vi "Helium Fridge Cool-Down.vi"() -> ()   [LabVIEW 2014]
uses:
  <vilib>/Analysis/8numeric.llb/1D Numeric Integration.vi
  <vilib>/express/express shared/transition.llb/Dynamic To Waveform Array.vi
  <vilib>/express/express signal manip/GetorSetDDTAttributes/Set DDT Attributes/SetT0.vi
  <vilib>/express/express shared/transition.llb/Waveform Array To Dynamic.vi
  <vilib>/express/express signal manip/GetorSetDDTAttributes/Set DDT Attributes/Set DDT Properties.xnode
  <vilib>/Analysis/NI_AALPro.lvlib
panel:
  in  "Submit":bool
  out "Is Flashing":bool
  in  "Error Beat":bool
  in  "Clear":bool
  in  "Comment":string
  out "Heartbeat":bool
  out "Most Recent Error":string
  out "Baseline Subtracted Integral vs. Time":dbl(graph)
  out "Time of Last Baseline":string
  out "Baseline":dbl[](array[numeric])
  in  "Baseline Subtract":bool
  in  "Get Baseline":bool
  out "Recording":bool
  out "Time of Last Recording":string
  in  "Record \nNMR Sweeps":bool
  in  "Depth/Div\n(kHz)":dbl=10.0
  in  "Central Freq. \n(MHz)":dbl=13.0
  in  "stop (F)":bool caption="Triangle Wave"
  in  "Triangle Wave\nRate (Hz)":dbl=0.3
  out "Time Elapsed \nDuring Sweeps (s)":dbl
  out "Lab Time":string
  out "Most Recent Error (NMR)":string
  out "Last Sweep Start Time":string
  out "Most Recent Error (Temp)":string
  out "Last Measurement Taken":string
  out "VI Start Time":string
  in  "Time Between\nTemp Ponts (s)":dbl=30.0
  out "Temp":bool
  out "NMR":bool
  in  "stop":bool
  out "Input Triangle Wave":dynamicdata(graph)
  out "Modulator":dynamicdata(graph)
  out "NMR":cluster{"Y":dbl[], "Y":dbl[]}[](graph)
  in  "# of Sweeps":dbl=1.0
  out "Resistance Strip Chart":dynamicdata(graph)
  out "Temperature Strip Chart":dynamicdata(graph)
  in  "Heartbeat":bool
  in  "Temp Strip Chart":bool
  out "Errors":bool
  in  "Silence Flashing":bool
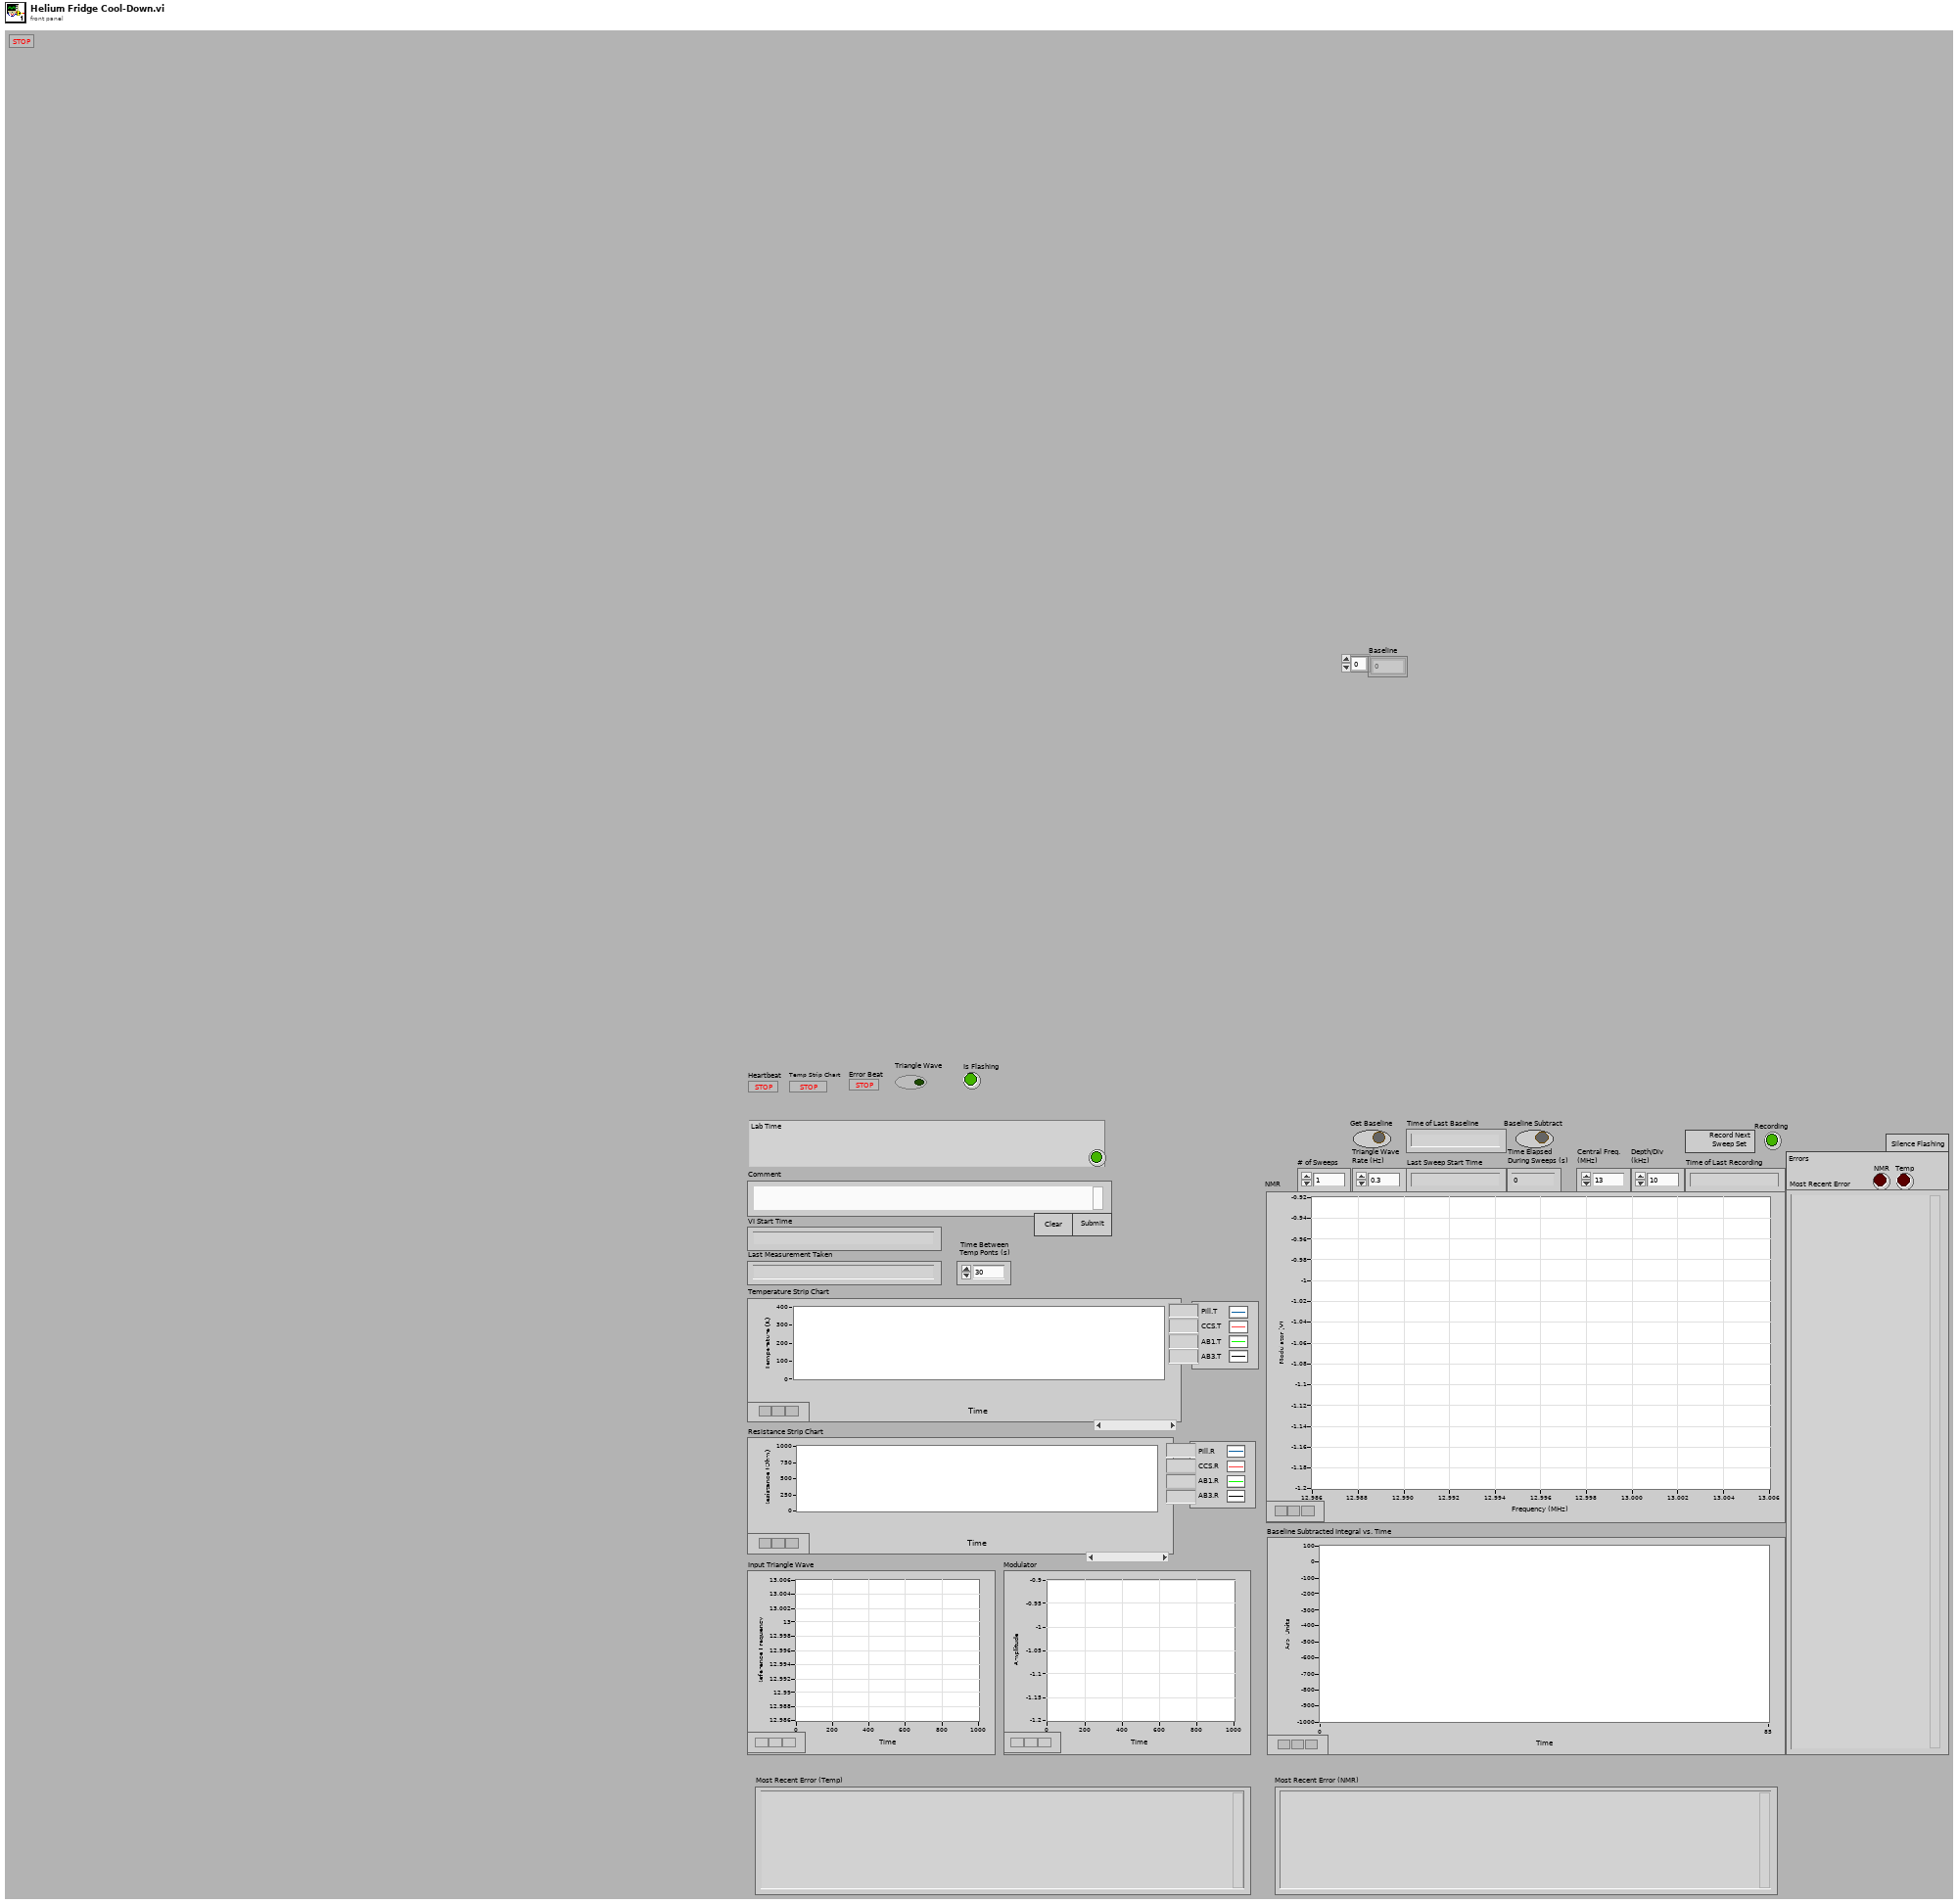
[diagram p1: front panel]
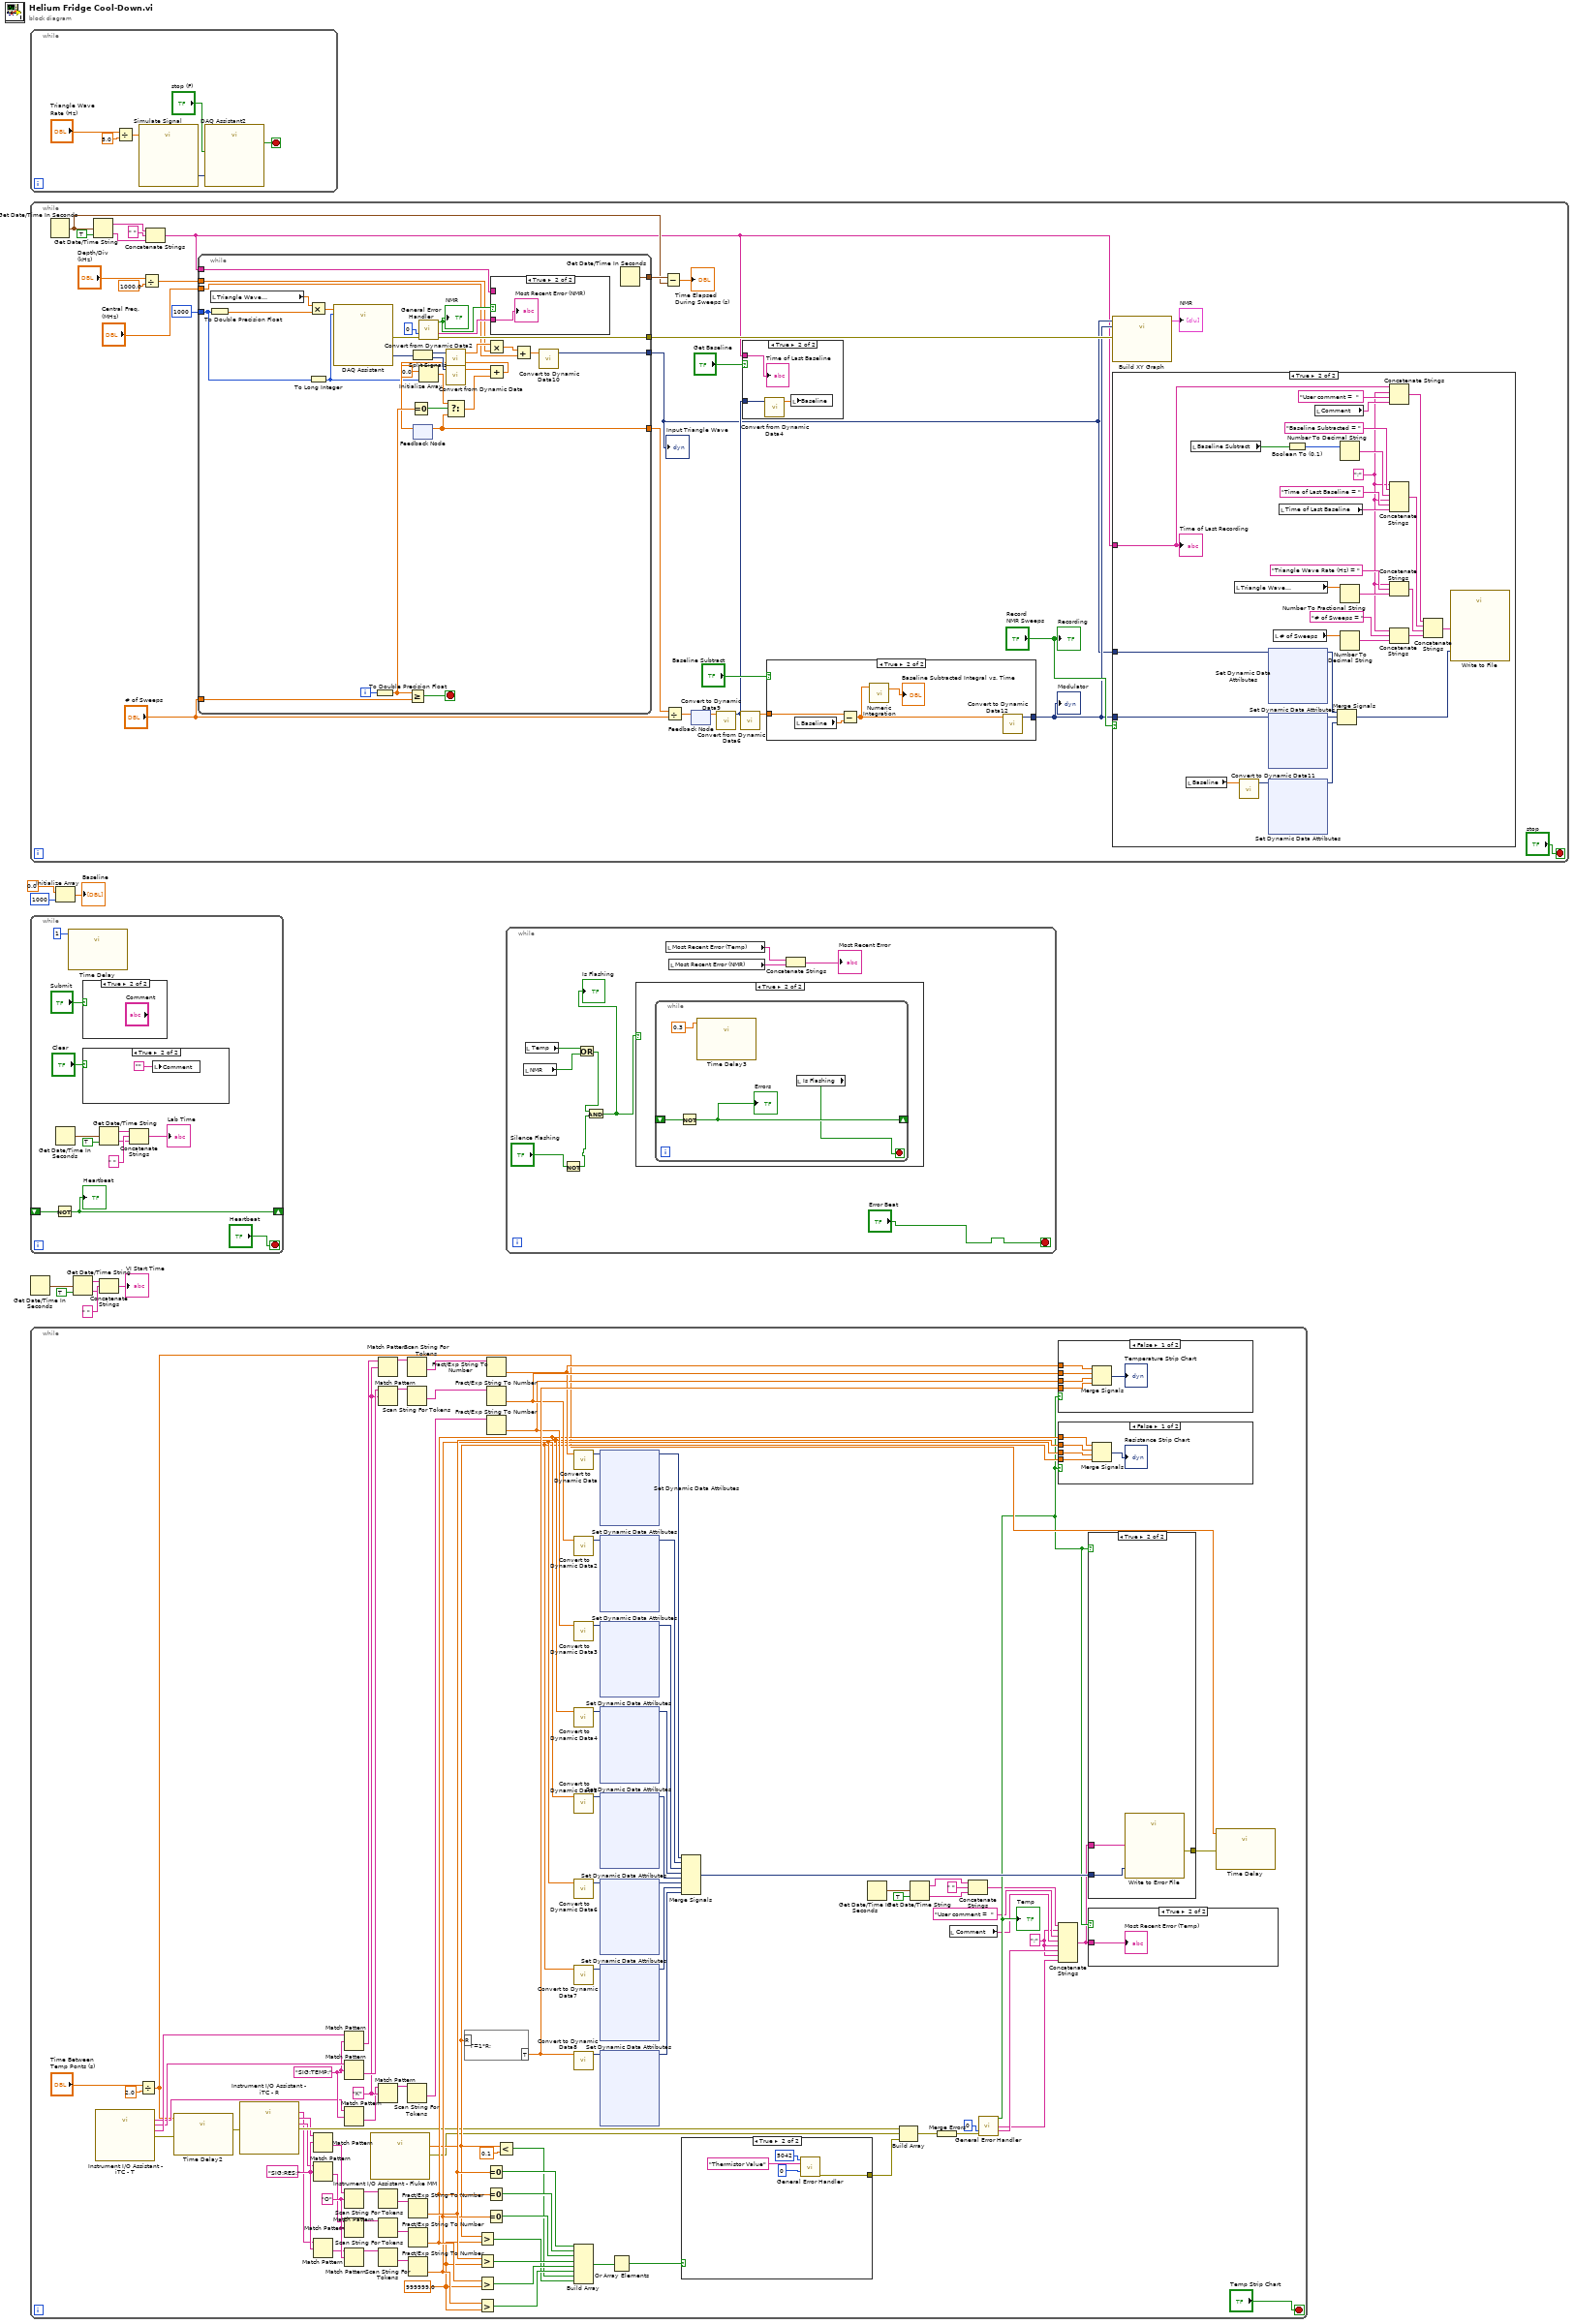
[diagram p0: block diagram]
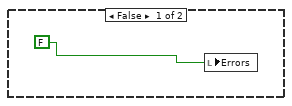
[diagram p2: hidden frame]
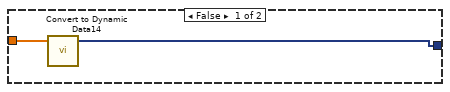
[diagram p3: hidden frame]
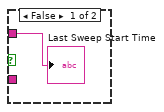
[diagram p6: hidden frame]
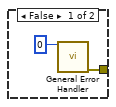
[diagram p9: hidden frame]
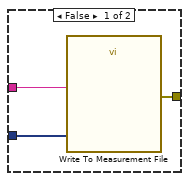
[diagram p12: hidden frame]
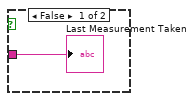
[diagram p13: hidden frame]
diagram:
  n1 = while {
    stop <- w14 stop-if-true
    n2 = Divide(x="Triangle Wave\nRate (Hz)", y=5.0) -> (x/y=w10:dbl)
    n3 = call "Simulate Signal"("Frequency"=w10) -> ("Triangle"=w13:dynamicdata)  [unwired: 13 in, 1 out]
    n4 = call "DAQ Assistant2"("data"=w13, "stop (F)"="stop (F)") -> ("stopped"=w14:bool)  [unwired: 15 in, 2 out]
  }
  n5 = while {
    stop <- "stop" stop-if-true
    n6 = Get Date/Time In Seconds() -> (seconds since 1Jan1904=w30:timestamp)
    n7 = Get Date/Time String(seconds (now)=w30, want seconds? (F)=TRUE) -> (date string=w33:string, time string=w35:string)  [unwired: 1 in]
    n8 = Divide(x="Depth/Div\n(kHz)", y=1000.0) -> (x/y=w24:dbl)
    n9 = Concatenate Strings(w33, " ", w35) -> (w16:string)
    n10 = while {
      tunnel: "# of Sweeps" -> [w163]
      tunnel: 1000 -> [w143]
      tunnel: [w156] -> w39
      tunnel: w16 -> [w150]
      tunnel: [w149] -> w31
      tunnel: [w147] -> w28
      tunnel: w24 -> [w140]
      tunnel: "Central Freq. \n(MHz)" -> [w138]
      tunnel: [w136] -> w17
      i -> [w164]
      stop <- w155 stop-if-true
      n11 = To Double Precision Float(number=w143) -> (double precision float=w144:dbl)
      n12 = local read "Triangle Wave\nRate (Hz)"() -> (w146:dbl)
      n13 = Multiply(x=w146, y=w144) -> (x*y=w148:dbl)
      n14 = To Long Integer(number=w143) -> (32bit integer=w145:i32)
      n15 = call "DAQ Assistant"("rate"=w148, "number of samples"=w145) -> ("data"=w166:dynamicdata, "error out"=w153:errorcluster)  [unwired: 15 in, 1 out]
      n16 = To Double Precision Float(number=w164) -> (double precision float=w162:dbl)
      n17 = Greater Or Equal?(x=w162, y=w163) -> (x >= y?=w155:bool)
      n18 = Equal To 0?(x=w162) -> (x = 0?=w161:bool)
      n19 = Split Signals(w166) -> (w142:dynamicdata, w165:dynamicdata)  [unwired: 2 in]
      n20 = feedback #1() -> (w156:dbl[])  [unwired: 1 in]
      n21 = call <vilib>:"General Error Handler.vi"("type of dialog (OK msg:1)"=0, "error in (no error)"=w153) -> ("error?"=w151:bool, "message"=w154:string, "error out"=w147:errorcluster)  [unwired: 9 in, 2 out]
      "NMR" <- w151
      n22 = Initialize Array(0.0, w145) -> (w159:dbl[])
      n23 = call "Convert from Dynamic Data2"("Dynamic Data Type"=w142) -> ("Array"=w141:dbl[])  [unwired: 3 in]
      n24 = call "Convert from Dynamic Data"("Dynamic Data Type"=w165) -> ("Array"=w158:dbl[])  [unwired: 3 in]
      n25 = Select(t=w159, s=w161, f=w156) -> (s? t:f=w160:dbl[])
      n26 = Multiply(x=w141, y=w140) -> (x*y=w139:dbl[])
      n27 = Add(x=w158, y=w160) -> (x+y=w157:dbl[])
      n28 = feedback-in #1(w157) -> ()
      n29 = case shown="True" w151 {
        tunnel: w154 -> [_ w169]
        tunnel: w150 -> [w168 _]
        frame False {
          "Last Sweep Start Time" <- w168
        }
        frame True {
          "Most Recent Error (NMR)" <- w169
        }
      }
      n30 = Add(x=w139, y=w138) -> (x+y=w137:dbl[])
      n31 = call "Convert to Dynamic Data10"("Array"=w137) -> ("Dynamic Data Type"=w136:dynamicdata)  [unwired: 3 in]
      n32 = Get Date/Time In Seconds() -> (seconds since 1Jan1904=w149:timestamp)
    }
    "Input Triangle Wave" <- w17
    n33 = Subtract(x=w31, y=w30) -> (x-y=→"Time Elapsed \nDuring Sweeps (s)":dbl)
    n34 = Divide(x=w39, y="# of Sweeps") -> (x/y=w37:dbl[])
    n35 = feedback-in #2(w37) -> ()
    n36 = feedback #2() -> (w36:dbl[])  [unwired: 1 in]
    n37 = call "Convert to Dynamic Data9"("Array"=w36) -> ("Dynamic Data Type"=w20:dynamicdata)  [unwired: 3 in]
    n38 = call "Convert from Dynamic Data6"("Dynamic Data Type"=w20) -> ("Array"=w19:dbl[])  [unwired: 3 in]
    n39 = case shown="True" "Get Baseline" {
      tunnel: w20 -> [_ w52]
      tunnel: w16 -> [_ w50]
      frame False {
      }
      frame True {
        n40 = call "Convert from Dynamic Data4"("Dynamic Data Type"=w52) -> ("Array"=w51:dbl[])  [unwired: 3 in]
        n41 = local write "Baseline"(w51) -> ()
        "Time of Last Baseline" <- w50
      }
    }
    n42 = case shown="True" "Baseline Subtract" {
      tunnel: w19 -> [w44 w49]
      tunnel: [w43 w48] -> w18
      frame False {
        n43 = call "Convert to Dynamic Data14"("Array"=w44) -> ("Dynamic Data Type"=w43:dynamicdata)  [unwired: 3 in]
      }
      frame True {
        n44 = local read "Baseline"() -> (w47:dbl[])
        n45 = Subtract(x=w49, y=w47) -> (x-y=w46:dbl[])
        n46 = call-poly <vilib>:"Numeric Integration.vi"("Input Array"=w46) -> ("result"=→"Baseline Subtracted Integral vs. Time":dbl)  [unwired: 2 in, 1 out]
        n47 = call "Convert to Dynamic Data12"("Array"=w46) -> ("Dynamic Data Type"=w48:dynamicdata)  [unwired: 3 in]
      }
    }
    "Modulator" <- w18
    n48 = call "Build XY Graph"("error in (no error)"=w28, "Y Input"=w18, "X Input"=w17) -> ("XY Graph"=→"NMR":cluster{"Y":dbl[], "Y":dbl[]}[])  [unwired: 7 in, 1 out]
    n49 = case shown="True" "Record \nNMR Sweeps" {
      tunnel: w16 -> [_ w69]
      tunnel: w18 -> [_ w77]
      tunnel: w17 -> [_ w76]
      frame False {
      }
      frame True {
        w53 = ";"
        n50 = local read "Baseline"() -> (w75:dbl[])
        n51 = local read "Baseline Subtract"() -> (w71:bool)
        n52 = local read "Triangle Wave\nRate (Hz)"() -> (w72:dbl)
        n53 = call "Convert to Dynamic Data11"("Array"=w75) -> ("Dynamic Data Type"=w74:dynamicdata)  [unwired: 3 in]
        n54 = xnode "Set Dynamic Data Attributes"("Signals In"=w76) -> ("Signals Out"=w81:dynamicdata)  [unwired: 4 in, 1 out]
        n55 = xnode "Set Dynamic Data Attributes"("Signals In"=w77) -> ("Signals Out"=w79:dynamicdata)  [unwired: 4 in, 1 out]
        n56 = xnode "Set Dynamic Data Attributes"("Signals In"=w74) -> ("Signals Out"=w73:dynamicdata)  [unwired: 4 in, 1 out]
        n57 = local read "# of Sweeps"() -> (w78:dbl)
        n58 = local read "Time of Last Baseline"() -> (w58:string)
        n59 = Boolean To (0,1)(Boolean=w71) -> (0, 1=w70:i16)
        n60 = local read "Comment"() -> (w67:string)
        n61 = Merge Signals(w81, w79, w73) -> (w80:dynamicdata)
        n62 = Number To Decimal String(number=w70) -> (decimal integer string=w63:string)  [unwired: 1 in]
        n63 = Number To Fractional String(number=w72) -> (F-format string=w61:string)  [unwired: 3 in]
        n64 = Number To Decimal String(number=w78) -> (decimal integer string=w65:string)  [unwired: 1 in]
        n65 = Concatenate Strings(w69, w53, "User comment =  ", w67) -> (w60:string)
        n66 = Concatenate Strings(w53, "Baseline Subtracted = ", w63, w53, "Time of Last Baseline = ", w58) -> (w57:string)
        n67 = Concatenate Strings(w53, "Triangle Wave Rate (Hz) = ", w61) -> (w56:string)
        n68 = Concatenate Strings(w53, "# of Sweeps = ", w65) -> (w55:string)
        n69 = Concatenate Strings(w60, w57, w56, w55) -> (w54:string)
        n70 = call "Write to File"("Signals"=w80, "Comment"=w54) -> ()  [unwired: 15 in, 3 out]
        "Time of Last Recording" <- w69
      }
    }
    "Recording" <- "Record \nNMR Sweeps"
  }
  n71 = while {
    shift-right: [w178] -> _
    shift-left: _ -> [w181]
    stop <- "Heartbeat" stop-if-true
    n72 = Not(x=w181) -> (.not. x?=w178:bool)
    "Heartbeat" <- w178
    n73 = Get Date/Time In Seconds() -> (seconds since 1Jan1904=w176:timestamp)
    n74 = call "Time Delay"("Delay Time (s)"=1) -> ()  [unwired: 10 in, 1 out]
    n75 = case shown="True" "Submit" {
      frame False {
      }
      frame True {
      }
    }
    n76 = case shown="True" "Clear" {
      frame False {
      }
      frame True {
        n77 = local write "Comment"("") -> ()
      }
    }
    n78 = Get Date/Time String(seconds (now)=w176, want seconds? (F)=TRUE) -> (date string=w175:string, time string=w173:string)  [unwired: 1 in]
    n79 = Concatenate Strings(w175, " ", w173) -> (→"Lab Time":string)
  }
  n80 = Get Date/Time In Seconds() -> (seconds since 1Jan1904=w8:timestamp)
  n81 = while {
    stop <- "Temp Strip Chart" stop-if-true
    w183 = ";"
    w207 = 999999.0
    w243 = "O"
    w244 = "SIG:RES:"
    w250 = "SIG:TEMP:"
    w249 = "K"
    n82 = call "Instrument I/O Assistant - iTC - T"() -> ("AB1.T"=w248:string, "CCS.T"=w253:string, "Pill.T"=w256:string, "error out"=w197:errorcluster)  [unwired: 23 in, 1 out]
    n83 = Divide(x="Time Between\nTemp Ponts (s)", y=2.0) -> (x/y=w192:dbl)
    n84 = call "Time Delay2"("error in (no error)"=w197, "Delay Time (s)"=w192) -> ("error out"=w198:errorcluster)  [unwired: 9 in]
    n85 = call "Instrument I/O Assistant - iTC - R"("error in"=w198) -> ("AB1.R"=w194:string, "CCS.R"=w195:string, "Pill.R"=w196:string, "error out"=w199:errorcluster)  [unwired: 22 in, 1 out]
    n86 = Match Pattern(string=w195, regular expression=w244) -> (after substring=w242:string)  [unwired: 1 in, 3 out]
    n87 = Match Pattern(string=w196, regular expression=w244) -> (after substring=w241:string)  [unwired: 1 in, 3 out]
    n88 = Match Pattern(string=w194, regular expression=w244) -> (after substring=w240:string)  [unwired: 1 in, 3 out]
    n89 = Match Pattern(string=w256, regular expression=w250) -> (after substring=w255:string)  [unwired: 1 in, 3 out]
    n90 = Match Pattern(string=w253, regular expression=w250) -> (after substring=w252:string)  [unwired: 1 in, 3 out]
    n91 = Match Pattern(string=w248, regular expression=w250) -> (after substring=w247:string)  [unwired: 1 in, 3 out]
    n92 = Match Pattern(string=w242, regular expression=w243) -> (before substring=w239:string)  [unwired: 1 in, 3 out]
    n93 = Match Pattern(string=w241, regular expression=w243) -> (before substring=w238:string)  [unwired: 1 in, 3 out]
    n94 = Match Pattern(string=w240, regular expression=w243) -> (before substring=w237:string)  [unwired: 1 in, 3 out]
    n95 = call "Instrument I/O Assistant - Fluke MM"() -> ("AB3.R"=w205:dbl, "error out"=w202:errorcluster)  [unwired: 25 in, 1 out]
    n96 = Match Pattern(string=w255, regular expression=w249) -> (before substring=w254:string)  [unwired: 1 in, 3 out]
    n97 = Match Pattern(string=w252, regular expression=w249) -> (before substring=w251:string)  [unwired: 1 in, 3 out]
    n98 = Match Pattern(string=w247, regular expression=w249) -> (before substring=w246:string)  [unwired: 1 in, 3 out]
    n99 = Scan String For Tokens(9:w239) -> (1:w236:string)  [unwired: 5 in, 3 out]
    n100 = Scan String For Tokens(9:w238) -> (1:w235:string)  [unwired: 5 in, 3 out]
    n101 = Scan String For Tokens(9:w237) -> (1:w234:string)  [unwired: 5 in, 3 out]
    n102 = Scan String For Tokens(9:w254) -> (1:w273:string)  [unwired: 5 in, 3 out]
    n103 = Scan String For Tokens(9:w251) -> (1:w271:string)  [unwired: 5 in, 3 out]
    n104 = Scan String For Tokens(9:w246) -> (1:w270:string)  [unwired: 5 in, 3 out]
    n105 = Fract/Exp String To Number(string=w236) -> (number=w213:dbl)  [unwired: 3 in, 1 out]
    n106 = Fract/Exp String To Number(string=w235) -> (number=w212:dbl)  [unwired: 3 in, 1 out]
    n107 = Fract/Exp String To Number(string=w234) -> (number=w211:dbl)  [unwired: 3 in, 1 out]
    n108 = formula code="T=1*R;"("R"=w205) -> ("T"=w224:dbl)
    n109 = Greater?(x=w205, y=w207) -> (0:w206:bool)
    n110 = Greater?(x=w213, y=w207) -> (0:w210:bool)
    n111 = Greater?(x=w212, y=w207) -> (0:w209:bool)
    n112 = Greater?(x=w211, y=w207) -> (0:w208:bool)
    n113 = Fract/Exp String To Number(string=w273) -> (number=w215:dbl)  [unwired: 3 in, 1 out]
    n114 = Fract/Exp String To Number(string=w271) -> (number=w216:dbl)  [unwired: 3 in, 1 out]
    n115 = Fract/Exp String To Number(string=w270) -> (number=w214:dbl)  [unwired: 3 in, 1 out]
    n116 = Equal To 0?(x=w213) -> (x = 0?=w221:bool)
    n117 = Equal To 0?(x=w212) -> (x = 0?=w220:bool)
    n118 = Equal To 0?(x=w211) -> (x = 0?=w219:bool)
    n119 = Less?(x=w205, y=0.1) -> (x < y?=w204:bool)
    n120 = Build Array(w221, w220, w219, w210, w209, w208, w204, w206) -> (w218:bool[])
    n121 = call "Convert to Dynamic Data"("Double"=w215) -> ("Dynamic Data Type"=w264:dynamicdata)  [unwired: 3 in]
    n122 = call "Convert to Dynamic Data2"("Double"=w216) -> ("Dynamic Data Type"=w262:dynamicdata)  [unwired: 3 in]
    n123 = call "Convert to Dynamic Data3"("Double"=w214) -> ("Dynamic Data Type"=w261:dynamicdata)  [unwired: 3 in]
    n124 = call "Convert to Dynamic Data4"("Double"=w213) -> ("Dynamic Data Type"=w233:dynamicdata)  [unwired: 3 in]
    n125 = call "Convert to Dynamic Data5"("Double"=w212) -> ("Dynamic Data Type"=w232:dynamicdata)  [unwired: 3 in]
    n126 = call "Convert to Dynamic Data6"("Double"=w211) -> ("Dynamic Data Type"=w231:dynamicdata)  [unwired: 3 in]
    n127 = call "Convert to Dynamic Data7"("Double"=w205) -> ("Dynamic Data Type"=w227:dynamicdata)  [unwired: 3 in]
    n128 = call "Convert to Dynamic Data8"("Double"=w224) -> ("Dynamic Data Type"=w223:dynamicdata)  [unwired: 3 in]
    n129 = xnode "Set Dynamic Data Attributes"("Signals In"=w264) -> ("Signals Out"=w263:dynamicdata)  [unwired: 4 in, 1 out]
    n130 = xnode "Set Dynamic Data Attributes"("Signals In"=w262) -> ("Signals Out"=w260:dynamicdata)  [unwired: 4 in, 1 out]
    n131 = xnode "Set Dynamic Data Attributes"("Signals In"=w261) -> ("Signals Out"=w259:dynamicdata)  [unwired: 4 in, 1 out]
    n132 = xnode "Set Dynamic Data Attributes"("Signals In"=w233) -> ("Signals Out"=w230:dynamicdata)  [unwired: 4 in, 1 out]
    n133 = xnode "Set Dynamic Data Attributes"("Signals In"=w232) -> ("Signals Out"=w229:dynamicdata)  [unwired: 4 in, 1 out]
    n134 = xnode "Set Dynamic Data Attributes"("Signals In"=w231) -> ("Signals Out"=w228:dynamicdata)  [unwired: 4 in, 1 out]
    n135 = xnode "Set Dynamic Data Attributes"("Signals In"=w227) -> ("Signals Out"=w226:dynamicdata)  [unwired: 4 in, 1 out]
    n136 = xnode "Set Dynamic Data Attributes"("Signals In"=w223) -> ("Signals Out"=w222:dynamicdata)  [unwired: 4 in, 1 out]
    n137 = Or Array Elements(Boolean array=w218) -> (logical OR=w217:bool)
    n138 = Merge Signals(w263, w260, w259, w230, w229, w228, w226, w222) -> (w258:dynamicdata)
    n139 = case shown="True" w217 {
      tunnel: [w274 w279] -> w201
      frame False {
        n140 = call <vilib>:"General Error Handler.vi"("[error code] (0)"=0) -> ("error out"=w274:errorcluster)  [unwired: 10 in, 4 out]
      }
      frame True {
        n141 = call <vilib>:"General Error Handler.vi"("[error code] (0)"=5042, "[error source] (\" \")"="Thermistor Value", "type of dialog (OK msg:1)"=0) -> ("error out"=w279:errorcluster)  [unwired: 8 in, 4 out]
      }
    }
    n142 = Get Date/Time In Seconds() -> (seconds since 1Jan1904=w269:timestamp)
    n143 = Build Array(w199, w202, w201) -> (w200:errorcluster[])
    n144 = Get Date/Time String(seconds (now)=w269, want seconds? (F)=TRUE) -> (date string=w267:string, time string=w265:string)  [unwired: 1 in]
    n145 = Merge Errors(w200) -> (w225:errorcluster)
    n146 = local read "Comment"() -> (w188:string)
    n147 = Concatenate Strings(w267, " ", w265) -> (w184:string)
    n148 = call <vilib>:"General Error Handler.vi"("type of dialog (OK msg:1)"=0, "error in (no error)"=w225) -> ("error?"=w191:bool, "source out"=w185:string, "message"=w187:string)  [unwired: 9 in, 2 out]
    "Temp" <- w191
    n149 = case shown="False" w191 {
      tunnel: w215 -> [w379 _]
      tunnel: w216 -> [w378 _]
      tunnel: w214 -> [w377 _]
      tunnel: w224 -> [w376 _]
      frame False {
        n150 = Merge Signals(w379, w378, w377, w376) -> (→"Temperature Strip Chart":dynamicdata)
      }
      frame True {
      }
    }
    n151 = case shown="False" w191 {
      tunnel: w212 -> [w374 _]
      tunnel: w213 -> [w373 _]
      tunnel: w211 -> [w372 _]
      tunnel: w205 -> [w371 _]
      frame False {
        n152 = Merge Signals(w374, w373, w372, w371) -> (→"Resistance Strip Chart":dynamicdata)
      }
      frame True {
      }
    }
    n153 = Concatenate Strings(w184, w183, "User comment =  ", w188, w183, w187, w183, w185) -> (w186:string)
    n154 = case shown="True" w191 {
      tunnel: w258 -> [w382 w385]
      tunnel: w186 -> [w381 w384]
      tunnel: [w380 w383] -> w245
      frame False {
        n155 = call "Write To Measurement File"("Signals"=w382, "Comment"=w381) -> ("error out"=w380:errorcluster)  [unwired: 15 in, 2 out]
      }
      frame True {
        n156 = call "Write to Error File"("Signals"=w385, "Comment"=w384) -> ("error out"=w383:errorcluster)  [unwired: 15 in, 2 out]
      }
    }
    n157 = case shown="True" w191 {
      tunnel: w186 -> [w440 w441]
      frame False {
        "Last Measurement Taken" <- w440
      }
      frame True {
        "Most Recent Error (Temp)" <- w441
      }
    }
    n158 = call "Time Delay"("error in (no error)"=w245, "Delay Time (s)"=w192) -> ()  [unwired: 9 in, 1 out]
  }
  n159 = Initialize Array(0.0, 1000) -> (→"Baseline":dbl[])
  n160 = Get Date/Time String(seconds (now)=w8, want seconds? (F)=TRUE) -> (date string=w7:string, time string=w5:string)  [unwired: 1 in]
  n161 = Concatenate Strings(w7, " ", w5) -> (→"VI Start Time":string)
  n162 = while {
    stop <- "Error Beat" stop-if-true
    n163 = local read "NMR"() -> (w450:bool)
    n164 = local read "Temp"() -> (w451:bool)
    n165 = Not(x="Silence Flashing") -> (.not. x?=w446:bool)
    n166 = Or(x=w451, y=w450) -> (x .or. y?=w448:bool)
    n167 = And(x=w448, y=w446) -> (x .and. y?=w445:bool)
    "Is Flashing" <- w445
    n168 = case shown="True" w445 {
      frame False {
        n169 = local write "Errors"(FALSE) -> ()
      }
      frame True {
        n170 = while {
          shift-right: [w454] -> _
          shift-left: _ -> [w456]
          stop <- w453 stop-if-true
          n171 = Not(x=w456) -> (.not. x?=w454:bool)
          "Errors" <- w454
          n172 = call "Time Delay3"("Delay Time (s)"=0.3) -> ()  [unwired: 10 in, 1 out]
          n173 = local read "Is Flashing"() -> (w453:bool)
        }
      }
    }
    n174 = local read "Most Recent Error (Temp)"() -> (w442:string)
    n175 = local read "Most Recent Error (NMR)"() -> (w443:string)
    n176 = Concatenate Strings(w442, w443) -> (→"Most Recent Error":string)
  }
